vi "Stimulus.Build.vi"(10 "CSVFile":path=path "C:/Denso FoDM Tester 2015/Denso-FoDM-Tester-2015/Continuous Monitoring Tester/Source/Project Files/VeriStand Project/Denso ELM/Sequences/Functional cycling 111715_Converted.CSV", 11 "StimulusPath":path=path "C:/Denso FoDM Tester 2015/Denso-FoDM-Tester-2015/Continuous Monitoring Tester/Source/Project Files/VeriStand Project/Denso ELM/Sequences/All.nivsstimprof") -> (0 "error out":errorcluster)   [LabVIEW 2015, in "RT Sequence Creation.lvlib"]
uses:
  NationalInstruments.VeriStand.RealTimeSequenceDefinitionApi
  RT Sequence Creation.lvlib
  Shared/Shared.lvlib
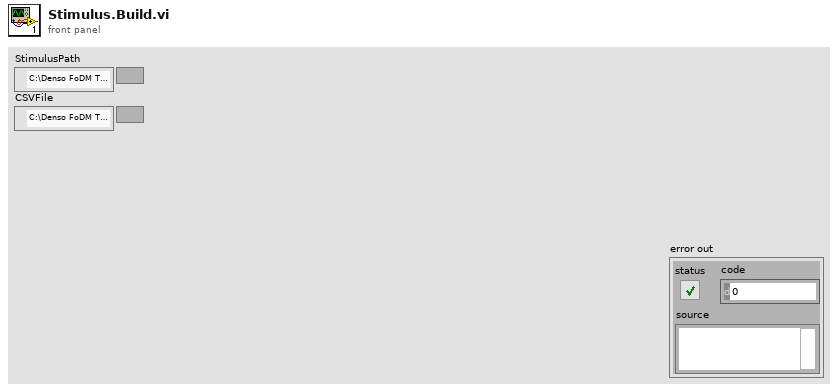
[diagram p1: front panel]
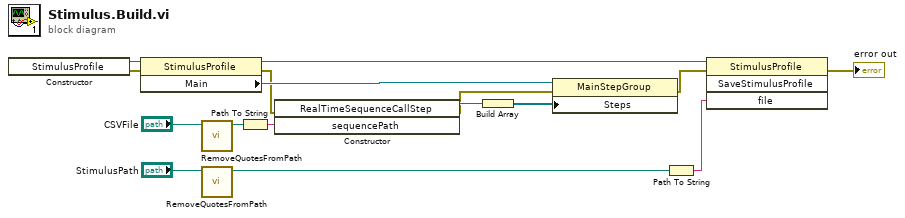
[diagram p0: block diagram]
diagram:
  n1 = constructor class="StimulusProfile"() -> (reference out=w16:refnum<k24>, error out=w15:errorcluster)  [unwired: 3 in, 1 out]
  n2 = property class="StimulusProfile"(reference=w16, error in=w15) -> (reference out=w12:refnum<k24>, error out=w7:errorcluster, "Main"=w13:refnum<k24>)
  n3 = call "RemoveQuotesFromPath.vi"("Data"="CSVFile") -> ("Path"=w1:path)  [unwired: 9 in, 1 out]
  n4 = call "RemoveQuotesFromPath.vi"("Data"="StimulusPath") -> ("Path"=w4:path)  [unwired: 9 in, 1 out]
  n5 = Path To String(path=w1) -> (string=w2:string)
  n6 = constructor class="RealTimeSequenceCallStep"(error in=w7, "sequencePath"=w2) -> (reference out=w11:refnum<k24>, error out=w6:errorcluster)  [unwired: 2 in, 2 out]
  n7 = Build Array(w11) -> (w10:refnum<k24>[])
  n8 = property class="MainStepGroup"(reference=w13, error in=w6, "Steps"=w10) -> (error out=w9:errorcluster)  [unwired: 1 out]
  n9 = Path To String(path=w4) -> (string=w14:string)
  n10 = invoke class="StimulusProfile" method="SaveStimulusProfile"(reference=w12, error in=w9, "file"=w14) -> (error out=→"error out":errorcluster)  [unwired: 1 in, 3 out]
